vi "Result Response.vi"(8 "error in (no error)":errorcluster, 10 "Acquired Result":refnum<class "Acquired Result.lvclass">, 11 "Measure Controller in":refnum<class "Process Controller.lvclass">) -> (0 "error out":errorcluster, 3 "Measure Controller out":refnum<class "Process Controller.lvclass">)   [LabVIEW 2016, in "Process Controller.lvclass"]
uses:
  Process Controller.lvclass
  C:/github/LabActor/Worker/Worker.lvclass
  NHMFL_Core/Libraries/Instruments/Results/Acquired Result/Acquired Result.lvclass
  Worker/Worker.lvclass/Worker.ctl
  Template Module/Read State.vi
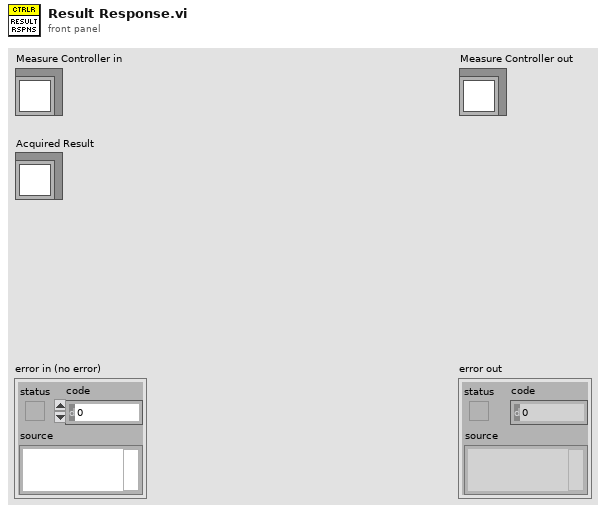
[diagram p1: front panel]
types:
  T1 = typedef "Worker State.ctl" = enum16{"Idle", "Starting", "Working", "Stopping"}
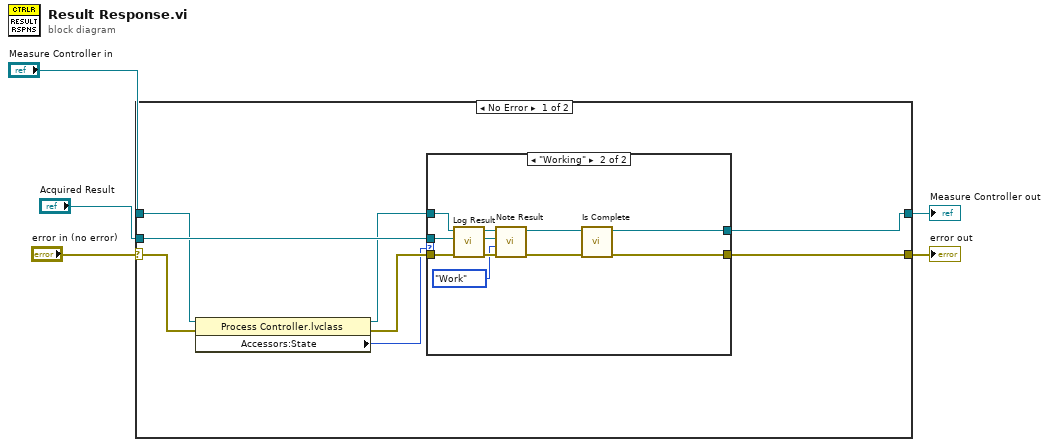
[diagram p0: block diagram]
diagram:
  n1 = case shown="No Error" "error in (no error)" {
    selector: "error in (no error)" -> [w8 w28]
    tunnel: [w12 w28] -> w4
    tunnel: [w13 w27] -> w2
    tunnel: "Measure Controller in" -> [w10 w27]
    tunnel: "Acquired Result" -> [w11 _]
    frame No Error {
      n2 = property class="Process Controller.lvclass"(reference=w10, error in=w8) -> (reference out=w9:refnum<class "Process Controller.lvclass">, error out=w7:errorcluster, "Accessors:State"=w6:T1)
      n3 = case shown="\"Working\"" w6 {
        tunnel: [w15 w26] -> w13
        tunnel: [w14 w25] -> w12
        tunnel: w11 -> [_ w20]
        tunnel: w9 -> [w15 w17]
        tunnel: w7 -> [w14 w16]
        frame "Idle", Default {
        }
        frame "Working" {
          n4 = call-dynamic "Log Result.vi"("error in (no error)"=w16, "Result"=w20, "Process Controller in"=w17) -> ("error out"=w21:errorcluster, "Result out"=w19:refnum<class "Acquired Result.lvclass">, "Process Controller out"=w22:refnum<class "Process Controller.lvclass">)  [unwired: 6 in]
          n5 = call-dynamic "Note Result.vi"("error in (no error)"=w21, "Stage"=enum16{"Init", "Work"}."Work", "Acquired Result.lvclass"=w19, "Measure Controller in"=w22) -> ("error out"=w23:errorcluster, "Measure Controller out"=w24:refnum<class "Process Controller.lvclass">)  [unwired: 6 in]
          n6 = call-dynamic "Is Complete.vi"("error in (no error)"=w23, "Measure Controller in"=w24) -> ("error out"=w25:errorcluster, "Measure Controller out"=w26:refnum<class "Process Controller.lvclass">)  [unwired: 8 in]
        }
      }
    }
    frame Error {
    }
  }
  "error out" <- w4
  "Measure Controller out" <- w2
